vi "Send Pre-Addressed Lock Publication.vi"(5 "PublicationPolicy":refnum<class "IPublicationPolicy.lvclass">, 6 "Return Error Transport":refnum<class "ITransport.lvclass">, 7 "Publisher ID":string, 8 "error in (no error)":errorcluster, 9 "Datum Type":variant, 10 "Datum Name":string, 11 "Lock Publication Msg":refnum<class "Lock Publication Msg.lvclass">) -> (0 "error out":errorcluster)   [LabVIEW 2020, in "IMediator.lvlib" / "Lock Publication Msg.lvclass"]
doc: "大多数想要发布数据的Actor或VI都会使用此send VI。调用此方法的Actor必须在发送之前收到预寻址的publish Msg。（对于Actor来说，这意味着它们是使用预寻址的发布消息启动的，或者是在中介激活后发送的。）"
uses:
  Lock Publication Msg.lvclass
  composed-transport/Source/ITransport/ITransport.lvclass
  IPublicationPolicy/IPublicationPolicy.lvclass
  Lock Publication Msg.lvclass/Lock Publication Msg.ctl
  composed-af-messages/Source/RoundTripMessage/RoundTripMessage.lvclass/RoundTripMessage.ctl
  <vilib>/ActorFramework/Message Enqueuer/Message Enqueuer.lvclass/Message Enqueuer.ctl
  <vilib>/ActorFramework/Message Enqueuer/Enqueue.vi
  composed-af-messages/Source/RoundTripMessage/RoundTripMessage.lvclass
  C:/Program Files/National Instruments/LabVIEW 2020/vi.lib/ActorFramework/Message/Message.lvclass
  <vilib>/ActorFramework/Message Priority Queue/Priority Enqueue.vi
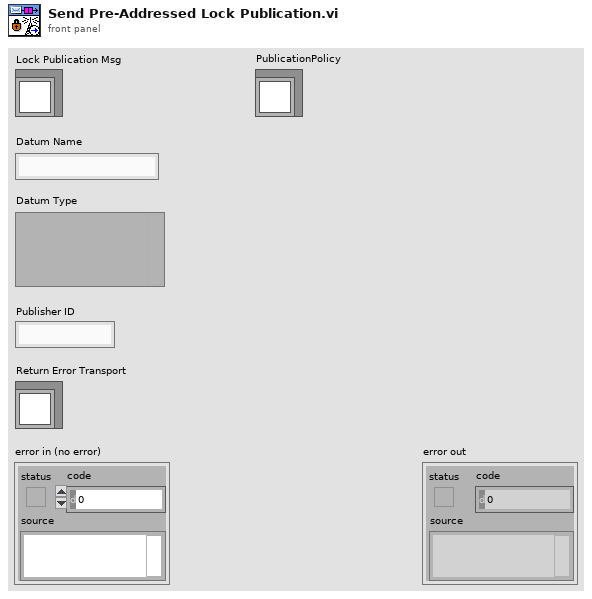
[diagram p1: front panel]
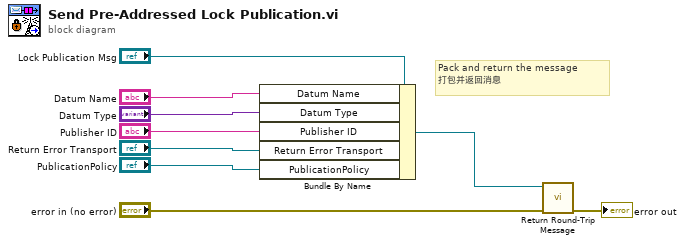
[diagram p0: block diagram]
diagram:
  # "Pack and return the message\n打包并返回消息"
  n1 = Bundle By Name(cluster="Lock Publication Msg", "Datum Name"="Datum Name", "Datum Type"="Datum Type", "Publisher ID"="Publisher ID", "Return Error Transport"="Return Error Transport", "PublicationPolicy"="PublicationPolicy") -> (w5:refnum<class "Lock Publication Msg.lvclass">)
  n2 = call "Return Round-Trip Message.vi"("error in (no error)"="error in (no error)", "RoundTripMessage In"=w5) -> ("error out"=→"error out":errorcluster)  [unwired: 9 in]
